vi "Buttons and diodes.vi"() -> ()   [LabVIEW 2012]
panel:
  out "data 2":dynamicdata(graph) caption="data"
  out "data":bool[](array[boolean])
  in  "stop":bool
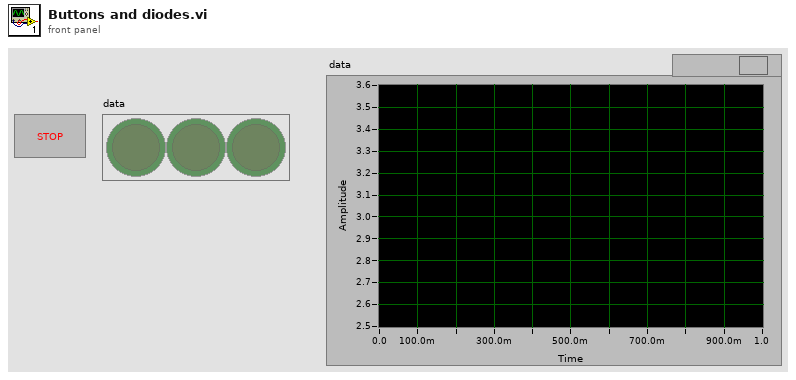
[diagram p1: front panel]
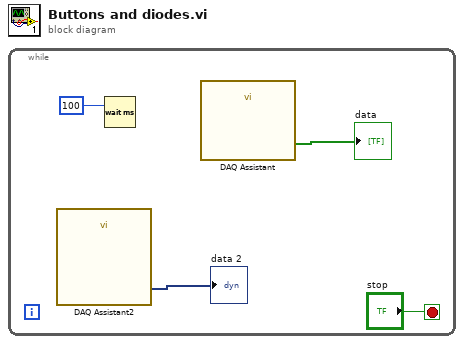
[diagram p0: block diagram]
diagram:
  n1 = while {
    stop <- "stop" stop-if-true
    n2 = call "DAQ Assistant2"() -> ("data"=→"data 2":dynamicdata)  [unwired: 17 in, 2 out]
    n3 = Wait (ms)(milliseconds to wait=100) -> ()  [unwired: 1 out]
    n4 = call "DAQ Assistant"() -> ("data"=→"data":bool[])  [unwired: 17 in, 2 out]
  }
